vi "Faults_v1.vi"(8 "error in":errorcluster caption="error in (no error)") -> (0 "error out":errorcluster, 2 "1D Array":dbl[](array[numeric]), 3 "2D Array":dbl[][](array[numeric]) format="%#_3g")   [LabVIEW 2022 SP3]
uses:
  <vilib>/DAQmx/write.llb/DAQmx Write (Digital 1D Bool NChan 1Samp 1Line).vi
  <vilib>/DAQmx/read.llb/DAQmx Read (Analog 1D DBL NChan 1Samp).vi
  <vilib>/DAQmx/miscellaneous.llb/DAQmx Fill In Error Info.vi
panel:
  # "GATEDRV_FLT_A"
  # "GATEDRV_FLT_B"
  # "GATEDRV_FLT_C"
  # "5V_A Fault"
  # "5V Fault"
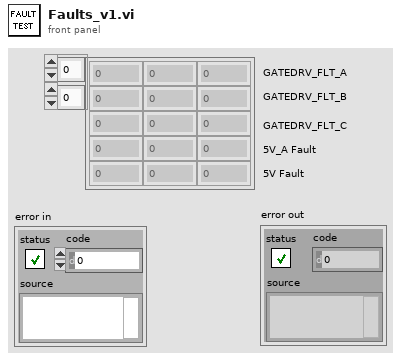
[diagram p1: front panel]
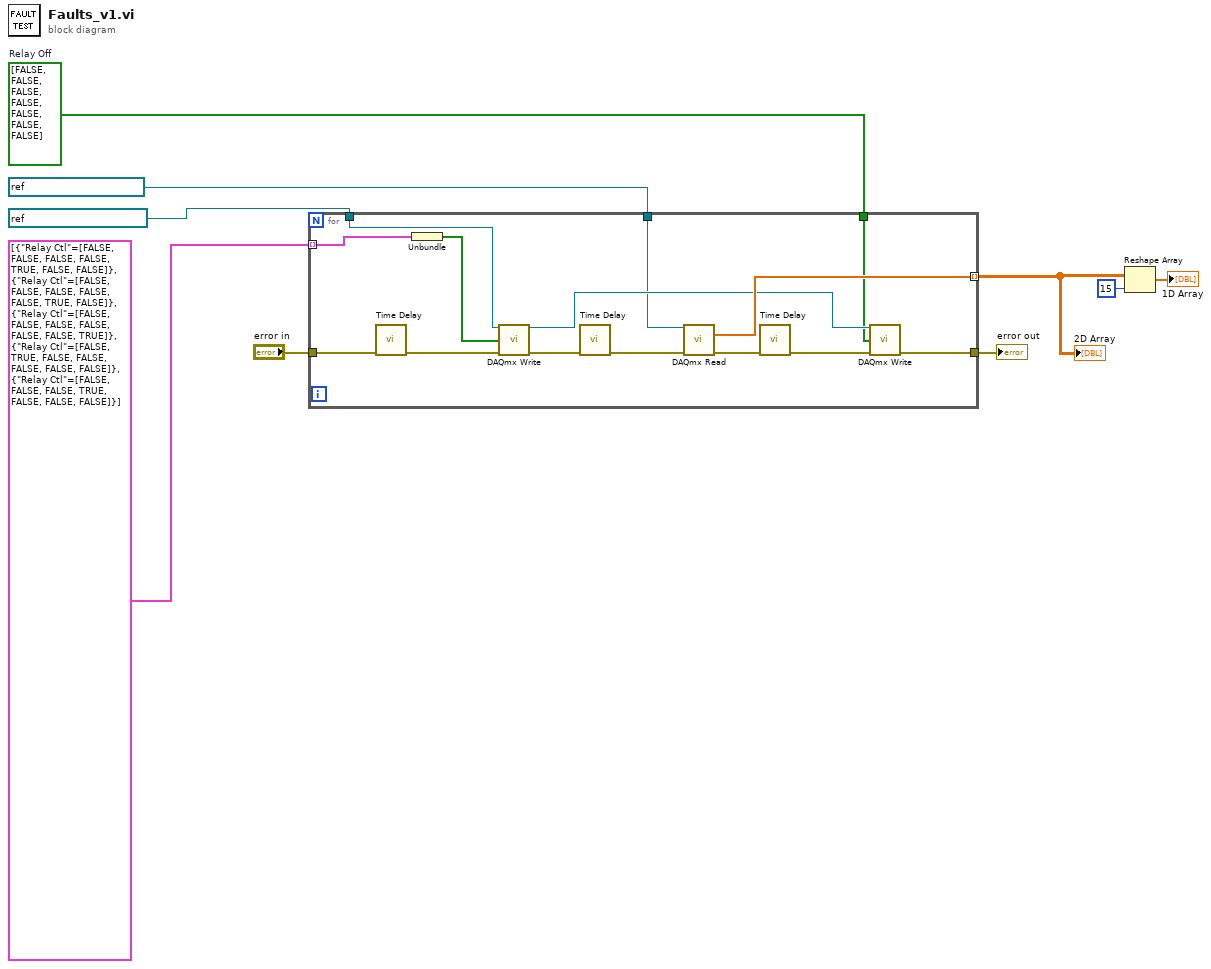
[diagram p0: block diagram]
diagram:
  w5 = bool[] [FALSE, FALSE, FALSE, FALSE, FALSE, FALSE, FALSE]  # Relay Off
  n1 = for {
    tunnel: cluster{"Relay Ctl":bool[]}[] [{"Relay Ctl"=[FALSE, FALSE, FALSE, FALSE, TRUE, FALSE, FALSE]}, {"Relay Ctl"=[FALSE, FALSE, FALSE, FALSE, FALSE, TRUE, FALSE]}, {"Relay Ctl"=[FALSE, FALSE, FALSE, FALSE, FALSE, FALSE, TRUE]}, {"Relay Ctl"=[FALSE, TRUE, FALSE, FALSE, FALSE, FALSE, FALSE]}, {"Relay Ctl"=[FALSE, FALSE, FALSE, TRUE, FALSE, FALSE, FALSE]}] -> [w23] mode=indexing
    tunnel: "error in" -> [w21]
    tunnel: [w18] -> w3 mode=indexing
    tunnel: [w15] -> w7
    tunnel: refnum<k21> "BONTS_Faults_Relays" ("task/channels in") -> [w12]
    tunnel: w5 -> [w11]
    tunnel: refnum<k21> "BONTS_Faults" ("task/channels in") -> [w10]
    n2 = call "Time Delay"("error in (no error)"=w21) -> ("error out"=w22:errorcluster)  [unwired: 10 in]
    n3 = Unbundle(w23) -> ("Relay Ctl"=w17:bool[])
    n4 = call-poly <vilib>:"DAQmx Write.vi"("task/channels in"=w12, "data"=w17, "error in"=w22) -> ("task out"=w13:refnum<k21>, "error out"=w20:errorcluster)  [unwired: 10 in, 1 out]
    n5 = call "Time Delay"("error in (no error)"=w20) -> ("error out"=w19:errorcluster)  [unwired: 10 in]
    n6 = call-poly <vilib>:"DAQmx Read.vi"("task/channels in"=w10, "error in"=w19) -> ("data"=w18:dbl[], "error out"=w16:errorcluster)  [unwired: 11 in, 1 out]
    n7 = call "Time Delay"("error in (no error)"=w16) -> ("error out"=w14:errorcluster)  [unwired: 10 in]
    n8 = call-poly <vilib>:"DAQmx Write.vi"("task/channels in"=w13, "data"=w11, "error in"=w14) -> ("error out"=w15:errorcluster)  [unwired: 10 in, 2 out]
  }
  "error out" <- w7
  "2D Array" <- w3
  n9 = Reshape Array(w3, 15 ("dimension size")) -> (→"1D Array":dbl[])
